vi "SeriellSchreiben.vi"(1 "Array 100*100 rgb":u32[][](array[colorbox]), 2 "Intensity 0-100":dbl(knob) min=0.0 max=100.0 step=1.0 scale=0.0..100.0, 3 "VISA resource name":refnum<visa-resource-name>) -> (0 "VISA resource name 2":refnum<visa-resource-name>)   [LabVIEW 2021]
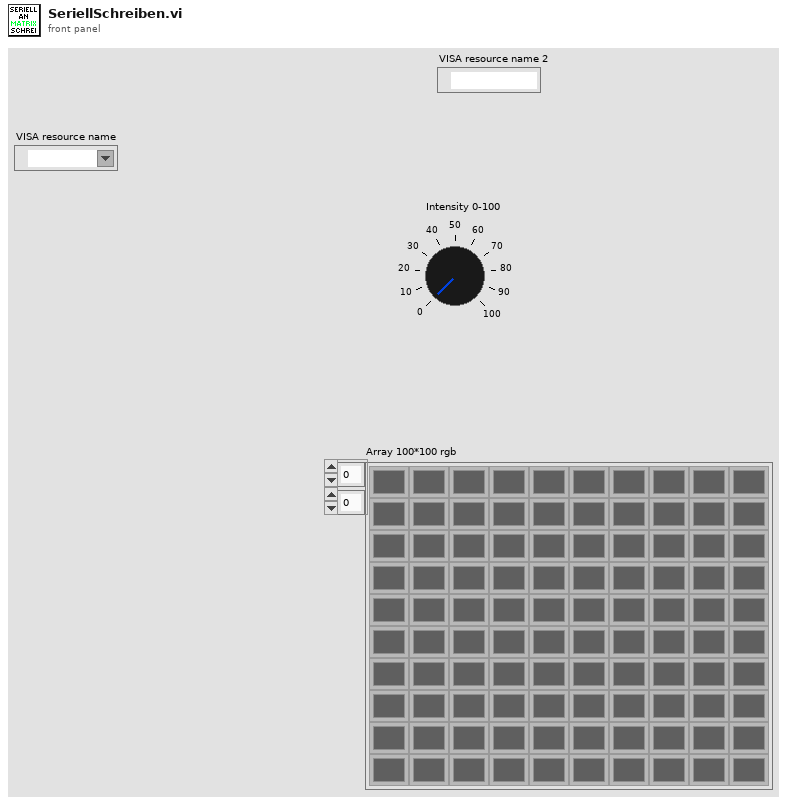
[diagram p1: front panel]
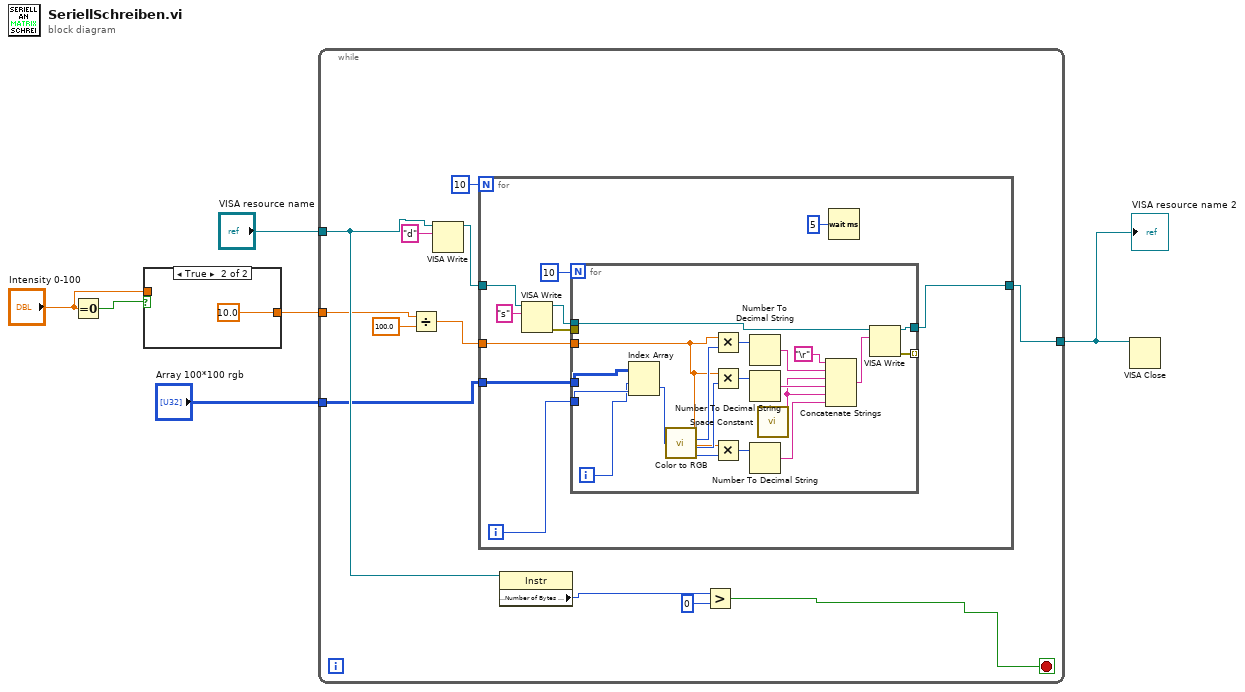
[diagram p0: block diagram]
diagram:
  n1 = Equal To 0?(x="Intensity 0-100") -> (x = 0?=w3:bool)
  n2 = case shown="True" w3 {
    tunnel: [w7 10.0 ("Intensity 0-100")] -> w2
    tunnel: "Intensity 0-100" -> [w7 _]
    frame False {
    }
    frame True {
    }
  }
  n3 = while {
    tunnel: [w20] -> w4
    tunnel: "VISA resource name" -> [w11]
    tunnel: "Array 100*100 rgb" -> [w10]
    tunnel: w2 -> [w9]
    stop <- w12 stop-if-true
    n4 = Divide(x=w9, y=100.0) -> (x/y=w18:dbl)
    n5 = VISA Write(VISA resource name=w11, write buffer="d") -> (VISA resource name out=w19:refnum<visa-resource-name>)  [unwired: 1 in, 2 out]
    n6 = for {
      N: 10 -> [_]
      tunnel: w10 -> [w28]
      tunnel: w18 -> [w27]
      tunnel: w19 -> [w26]
      tunnel: [w29] -> w20
      i -> [w23]
      n7 = VISA Write(VISA resource name=w26, write buffer="s") -> (VISA resource name out=w25:refnum<visa-resource-name>, error out=w21:errorcluster)  [unwired: 1 in, 1 out]
      n8 = for {
        N: 10 -> [_]
        tunnel: [w39] -> w29
        tunnel: w28 -> [w37]
        tunnel: w27 -> [w35]
        tunnel: w25 -> [w34]
        tunnel: w23 -> [w33]
        tunnel: w21 -> [_]
        tunnel: [w31] -> _ mode=indexing
        i -> [w32]
        n9 = Index Array(array=w37, index (row)=w32, index (col)=w33) -> (element=w36:u32)
        n10 = call <vilib>:"Color to RGB.vi"("Color"=w36) -> ("R"=w45:u8, "G"=w40:u8, "B"=w42:u8)  [unwired: 1 out]
        n11 = Multiply(x=w35, y=w45) -> (x*y=w44:u8)
        n12 = Multiply(x=w35, y=w40) -> (x*y=w41:u8)
        n13 = Multiply(x=w35, y=w42) -> (x*y=w43:u8)
        n14 = Number To Decimal String(number=w44) -> (decimal integer string=w50:string)  [unwired: 1 in]
        n15 = Number To Decimal String(number=w41) -> (decimal integer string=w49:string)  [unwired: 1 in]
        n16 = Number To Decimal String(number=w43) -> (decimal integer string=w48:string)  [unwired: 1 in]
        n17 = call <vilib>:"Space Constant.vi"() -> ("String"=w47:string)
        n18 = Concatenate Strings("\r", w50, w47, w49, w47, w48) -> (w38:string)
        n19 = VISA Write(VISA resource name=w34, write buffer=w38) -> (VISA resource name out=w39:refnum<visa-resource-name>, error out=w31:errorcluster)  [unwired: 1 in, 1 out]
      }
      n20 = Wait (ms)(milliseconds to wait=u32 5) -> ()  [unwired: 1 out]
    }
    n21 = property class="Instr"(reference=w11) -> ("Serial Settings:Number of Bytes at Serial Port"=w14:u32)  [unwired: 1 in, 2 out]
    n22 = Greater?(x=w14, y=u32 0) -> (0:w12:bool)
  }
  "VISA resource name 2" <- w4
  n23 = VISA Close(VISA resource name=w4) -> ()  [unwired: 1 in, 1 out]
